vi "Load Pictures.vi"() -> (0 "error out":errorcluster)   [LabVIEW 2020, in "VolatusGUIElements.lvlib" / "2WayValveH.lvclass"]
uses:
  2WayValveH.lvclass
  Picture.ctl
  2WayValveH.lvclass/2WayValveH.ctl
  volatus-gui-controls/VolatusGUIControls/VolatusGUIControls.lvlib
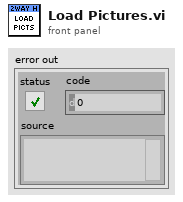
[diagram p1: front panel]
types:
  T1 = typedef "VolatusGUIElements.lvlib/2WayValveH.lvclass/Picture.ctl" = enum16{"Blank", "OutClose", "OutOpen", "OutTranClose", "OutTranOpen", "OutConfig", "OutStale", "OutError", "InClose", "InOpen", "InTranClose", "InTranOpen", "InConfig", "InStale", "InError", "EnOff", "EnOn", "EnConfig", "EnStale", "EnError"}
  T2 = typedef "imagedata.ctl" = cluster{"image type":i32, "image depth":i32, "image":u8[], "mask":u8[], "colors":u32[], "Rectangle":cluster{"left":i16, "top":i16, "right":i16, "bottom":i16}}
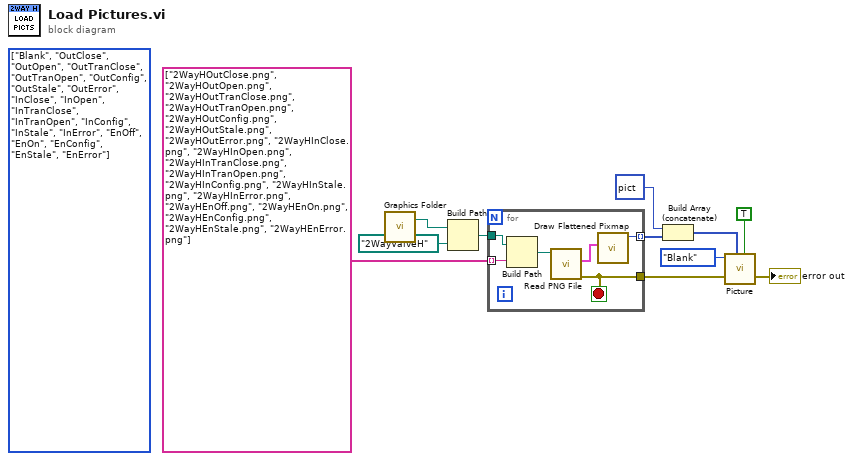
[diagram p0: block diagram]
diagram:
  (unwired) T1[] [enum."Blank", enum."OutClose", enum."OutOpen", enum."OutTranClose", enum."OutTranOpen", enum."OutConfig", enum."OutStale", enum."OutError", enum."InClose", enum."InOpen", enum."InTranClose", enum."InTranOpen", enum."InConfig", enum."InStale", enum."InError", enum."EnOff", enum."EnOn", enum."EnConfig", enum."EnStale", enum."EnError"] items=["Blank", "OutClose", "OutOpen", "OutTranClose", "OutTranOpen", "OutConfig", "OutStale", "OutError", "InClose", "InOpen", "InTranClose", "InTranOpen", "InConfig", "InStale", "InError", "EnOff", "EnOn", "EnConfig", "EnStale", "EnError"]
  n1 = call "Graphics Folder.vi"() -> ("Graphics Folder"=w2:path)  [unwired: 3 in]
  n2 = Build Path(base path=w2, name or relative path=path "2WayValveH") -> (appended path=w3:path)
  n3 = for {
    tunnel: w3 -> [w16]
    tunnel: string[] ["2WayHOutClose.png", "2WayHOutOpen.png", "2WayHOutTranClose.png", "2WayHOutTranOpen.png", "2WayHOutConfig.png", "2WayHOutStale.png", "2WayHOutError.png", "2WayHInClose.png", "2WayHInOpen.png", "2WayHInTranClose.png", "2WayHInTranOpen.png", "2WayHInConfig.png", "2WayHInStale.png", "2WayHInError.png", "2WayHEnOff.png", "2WayHEnOn.png", "2WayHEnConfig.png", "2WayHEnStale.png", "2WayHEnError.png"] -> [w15] mode=indexing
    tunnel: [w12] -> w7
    tunnel: [w11] -> w9 mode=indexing
    stop <- w12 stop-if-true
    n4 = Build Path(base path=w16, name or relative path=w15) -> (appended path=w14:path)
    n5 = call <vilib>:"Read PNG File.vi"("path to PNG file"=w14) -> ("error out"=w12:errorcluster, "image data"=w13:T2)  [unwired: 8 in, 1 out]
    n6 = call <vilib>:"Draw Flattened Pixmap.vi"("image data"=w13) -> ("new picture"=w11:picture)  [unwired: 8 in]
  }
  "error out" <- w7
  n7 = Build Array (concatenate)(picture data[5B] ("picture"), w9) -> (w5:picture[])
  n8 = call "Picture.vi"("Set Pictures (F)"=TRUE, "Pictures"=w5, "Picture Item"=Picture."Blank") -> ()  [unwired: 8 in, 1 out]
